vi "source_ramp_voltage.vi"(0 "Input parameters":T1={"Measurement type"=enum."Debug", "Sensor type"=enum."HPK_8in_256", "Identifier"="test.txt", "Open after execution?"=FALSE, "Plot after execution?"=FALSE, "Display channel"=0, "Voltage Delay (s)"=0.5, "Switch Delay (s)"=0.01, "VISA resource name source"="", "VISA resource name DMM"="", "VISA resource name LCR"="", "Compliance  Level (A)"=10.0, "Voltage Limit (V)"=1000.0, "Data storage location"="", "Scan voltages"="", "Use source as DMM?"=FALSE, "LCR signal frequenzy (Hz)"=10.0, "DMM device"=enum."Keithley2001", "Sampling number"=1, "Use env. sensors on"=enum."Sensirion sht1x/7x", "Switchboard Handle"=0, "Use Switchboard"=FALSE, "LCR signal voltage (V)"=10000.0, "Repeat"=1, "Scan voltages IV"="", "Scan voltages CV"="", "Hex pad numbers?"=FALSE, "Set measurement type"=enum."Debug", "Custom pad scan"="", "IV voltage Delay (s)"=0.5, "CV voltage Delay (s)"=0.5, "Needle measurement?"=FALSE, "Comments"="test.txt", "LCR signal frequenzy (kHz)"=10.0, "Compliance  Level (uA)"=10.0, "Open Correction Array"=array2304x3[6912 elements], "Current set voltage"=0.0, "Last set voltage"=0.0, "Current channel"=0, "Last OpenCorrection index"=-1, "Total curr/vltg every x steps"=10, "Current channel iteration"=0, "No CV corrections"=FALSE, "Mapfile"="", "Corrfile"="", "IV voltage file"=path "", "CV voltage file"=path "", "IV Switch Delay (s)"=0.01, "CV Switch Delay (s)"=0.01} {"CV Switch Delay (s)" format="%#_13g"; "IV Switch Delay (s)" format="%#_13g"; "Last set voltage" format="%#_13g"; "Current set voltage" format="%#_13g"; "CV voltage Delay (s)" format="%#_13g"; "IV voltage Delay (s)" format="%#_13g"; "Voltage Limit (V)" format="%#_13g"; "Voltage Delay (s)" format="%#_13g"; "Switch Delay (s)" format="%#_13g"}, 2 "Stop":refnum<vi>, 7 "Target voltage (V)":dbl, 9 "Compliance Current (A)":dbl=0.1, 11 "error in (no error)":errorcluster) -> (4 "VISA resource name out":refnum<visa-resource-name>, 6 "Current voltage out (V)":dbl, 8 "Aborted?":bool, 15 "error out":errorcluster)   [LabVIEW 2016]
uses:
  input_params.ctl
  <instrlib>/Keithley 24XX/Keithley 24XX.lvlib
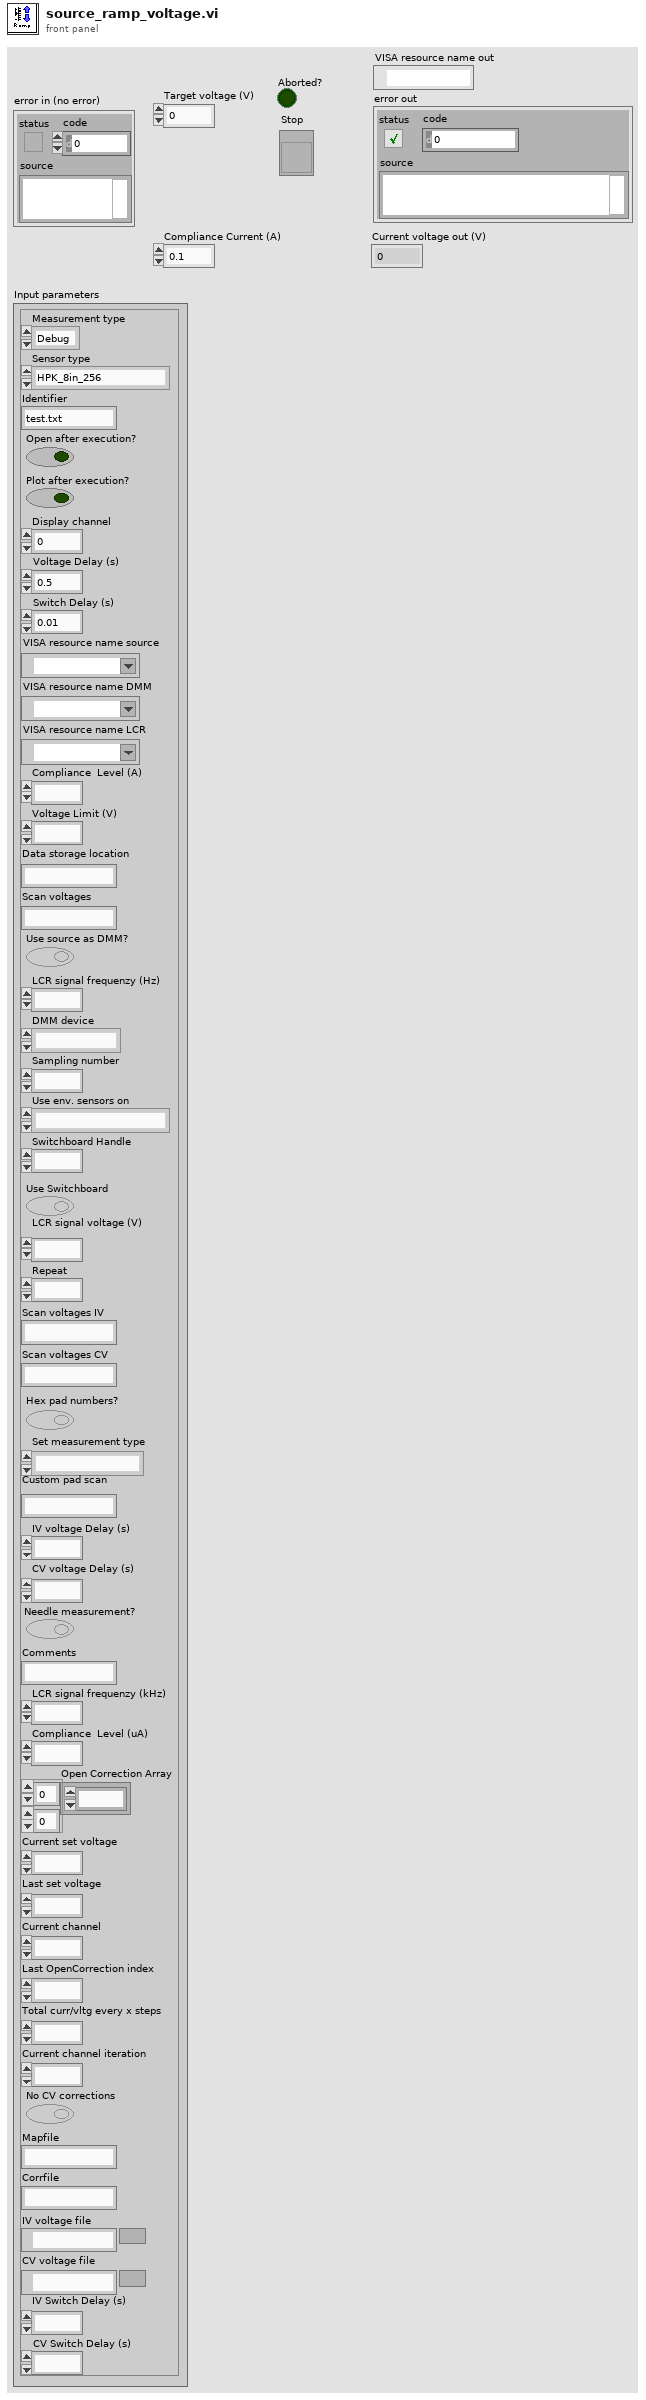
[diagram p1: front panel]
types:
  T1 = typedef "input_params.ctl" = cluster{"Measurement type":enum16{"IV", "CV", "Debug", "Test_contact"}, "Sensor type":enum16{"HPK_6in_135", "HPK_8in_256", "IFX_8in_256", "Diode", "HPK_6in_256", "Full matrix"}, "Identifier":string, "Open after execution?":bool, "Plot after execution?":bool, "Display channel":i32, "Voltage Delay (s)":dbl, "Switch Delay (s)":dbl, "VISA resource name source":refnum<visa-resource-name>, "VISA resource name DMM":refnum<visa-resource-name>, "VISA resource name LCR":refnum<visa-resource-name>, "Compliance  Level (A)":dbl, "Voltage Limit (V)":dbl, "Data storage location":string, "Scan voltages":string, "Use source as DMM?":bool, "LCR signal frequenzy (Hz)":dbl, "DMM device":enum16{"Keithley2001", "Keithley2450", "Keithley2410", "Keithley6487"}, "Sampling number":i32, "Use env. sensors on":enum16{"Sensirion sht1x/7x", "Switch Matrix", "Probecard"}, "Switchboard Handle":u32, "Use Switchboard":bool, "LCR signal voltage (V)":dbl, "Repeat":i32, "Scan voltages IV":string, "Scan voltages CV":string, "Hex pad numbers?":bool, "Set measurement type":enum16{"IV", "CV", "Debug", "Test_contact", "IV+CV"}, "Custom pad scan":string, "IV voltage Delay (s)":dbl, "CV voltage Delay (s)":dbl, "Needle measurement?":bool, "Comments":string, "LCR signal frequenzy (kHz)":dbl, "Compliance  Level (uA)":dbl, "Open Correction Array":dbl[][], "Current set voltage":dbl, "Last set voltage":dbl, "Current channel":i32, "Last OpenCorrection index":i32, "Total curr/vltg every x steps":i32, "Current channel iteration":i32, "No CV corrections":bool, "Mapfile":string, "Corrfile":string, "IV voltage file":path, "CV voltage file":path, "IV Switch Delay (s)":dbl, "CV Switch Delay (s)":dbl}
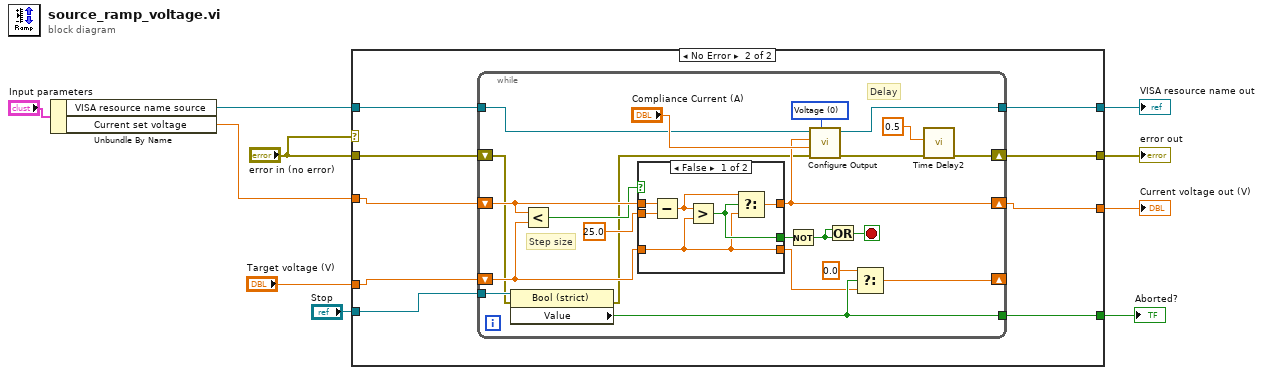
[diagram p0: block diagram]
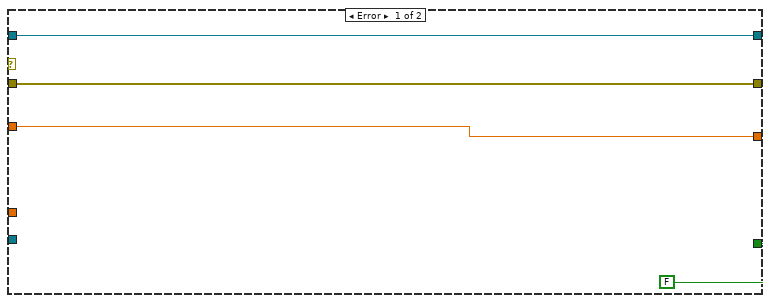
[diagram p2: hidden frame]
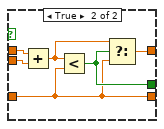
[diagram p3: hidden frame]
diagram:
  n1 = Unbundle By Name("Input parameters") -> ("VISA resource name source"=w2:refnum<visa-resource-name>, "Current set voltage"=w1:dbl)
  n2 = case shown="No Error" "error in (no error)" {
    tunnel: "error in (no error)" -> [w13 w23]
    tunnel: "Target voltage (V)" -> [_ w16]
    tunnel: w1 -> [w14 w17]
    tunnel: w2 -> [w12 w22]
    tunnel: [w12 w21] -> w9
    tunnel: [w13 w20] -> w8
    tunnel: [w14 w15] -> w7
    tunnel: "Stop" -> [_ w19]
    tunnel: [FALSE ("Value") w18] -> w4
    frame Error {
    }
    frame No Error {
      n3 = while {
        shift-right: [w31] -> w20
        shift-left: w23 -> [w25]
        shift-right: [w33] -> w15
        shift-left: w17 -> [w36]
        tunnel: w22 -> [w41]
        tunnel: [w30] -> w21
        tunnel: w19 -> [w37]
        shift-right: [w26] -> _
        shift-left: w16 -> [w35]
        tunnel: [w29] -> w18
        stop <- w40 stop-if-true
        w42 = u16 0 items=["Voltage", "Current"] ("Source Mode  (0: Voltage)")
        # "Delay"
        # "Step size"
        n4 = property class="Bool (strict)"(reference=w37, error in=w25) -> (error out=w24:errorcluster, "Value"=w29:bool)  [unwired: 1 out]
        n5 = Less?(x=w36, y=w35) -> (x < y?=w34:bool)
        n6 = case shown="False" w34 {
          tunnel: w35 -> [w46 w52]
          tunnel: 25.0 ("Step size (V)") -> [w50 w56]
          tunnel: w36 -> [w51 w57]
          tunnel: [w48 w54] -> w33
          tunnel: [w47 w53] -> w39
          tunnel: [w46 w52] -> w27
          frame False {
            n7 = Subtract(x=w51, y=w50) -> (x-y=w49:dbl)
            n8 = Greater?(x=w49, y=w46) -> (0:w47:bool)
            n9 = Select(t=w49, s=w47, f=w46) -> (s? t:f=w48:dbl)
          }
          frame True {
            n10 = Add(x=w57, y=w56) -> (x+y=w55:dbl)
            n11 = Less?(x=w55, y=w52) -> (x < y?=w53:bool)
            n12 = Select(t=w55, s=w53, f=w52) -> (s? t:f=w54:dbl)
          }
        }
        n13 = Not(x=w39) -> (.not. x?=w38:bool)
        n14 = call <instrlib>:"Configure Output.vi"("Source Mode  (0: Voltage)"=w42, "error in (no error)"=w24, "Compliance  Level (0.1)"="Compliance Current (A)", "Output Level (0)"=w33, "VISA resource name"=w41) -> ("error out"=w32:errorcluster, "VISA resource name out"=w30:refnum<visa-resource-name>)  [unwired: 5 in]
        n15 = Or(x=w38, y=w38) -> (x .or. y?=w40:bool)
        n16 = Select(t=0.0 ("Target voltage (V)"), s=w29, f=w27) -> (s? t:f=w26:dbl)
        n17 = call "Time Delay2"("error in (no error)"=w32, "Delay Time (s)"=0.5 ("Delay (s)")) -> ("error out"=w31:errorcluster)  [unwired: 9 in]
      }
    }
  }
  "VISA resource name out" <- w9
  "error out" <- w8
  "Current voltage out (V)" <- w7
  "Aborted?" <- w4
